vi "EXA_RBW.vi"(0 "VISA resource name":refnum<visa-resource-name>, 5 "Mode":enum16{"Set", "Get"}(ring), 7 "Units":enum16{"Hz", "kHz", "MHz", "GHz"}(ring), 9 "RBW":dbl, 11 "error in":errorcluster) -> (4 "VISA resource name":refnum<visa-resource-name>, 6 "RBW(Hz)":dbl, 15 "error out":errorcluster)   [LabVIEW 2016]
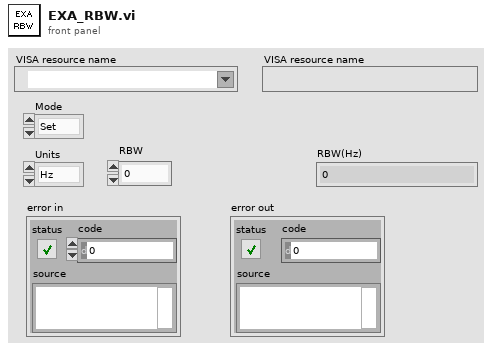
[diagram p1: front panel]
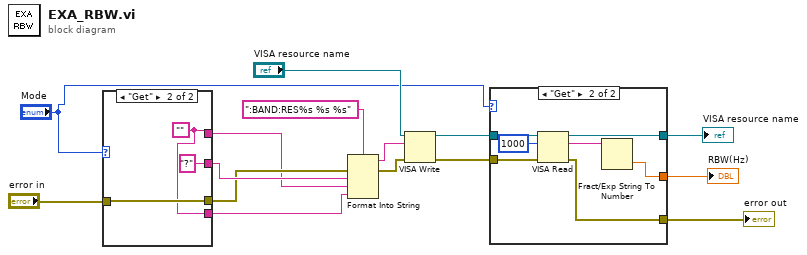
[diagram p0: block diagram]
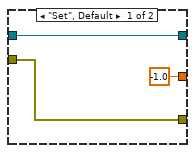
[diagram p2: hidden frame]
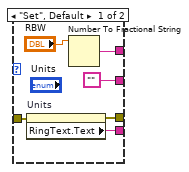
[diagram p3: hidden frame]
diagram:
  n1 = case shown="\"Get\"" "Mode" {
    tunnel: [w16 w22] -> w1
    tunnel: [w21 w22] -> w2
    tunnel: "error in" -> [w20 w23]
    tunnel: [w19 w23] -> w3
    tunnel: ["" "?"] -> w4
    frame "Set", Default {
      n2 = property on="Units" class="Enum (strict)"(error in=w20) -> (error out=w19:errorcluster, "RingText.Text"=w21:string)  [unwired: 1 in, 1 out]
      n3 = Number To Fractional String(number="RBW") -> (F-format string=w16:string)  [unwired: 3 in]
    }
    frame "Get" {
      w22 = ""
    }
  }
  n4 = Format Into String(format string=":BAND:RES%s %s %s", error in=w3, w4, w1, w2) -> (resulting string=w12:string, error out=w14:errorcluster)  [unwired: 1 in]
  n5 = VISA Write(VISA resource name="VISA resource name", write buffer=w12, error in (no error)=w14) -> (VISA resource name out=w8:refnum<visa-resource-name>, error out=w9:errorcluster)  [unwired: 1 out]
  n6 = case shown="\"Get\"" "Mode" {
    tunnel: w9 -> [w25 w34]
    tunnel: w8 -> [w27 w33]
    tunnel: [w27 w32] -> w5
    tunnel: [-1.0 w30] -> w7
    tunnel: [w25 w29] -> w6
    frame "Set", Default {
    }
    frame "Get" {
      n7 = VISA Read(VISA resource name=w33, byte count=u32 1000, error in (no error)=w34) -> (VISA resource name out=w32:refnum<visa-resource-name>, read buffer=w31:string, error out=w29:errorcluster)  [unwired: 1 out]
      n8 = Fract/Exp String To Number(string=w31) -> (number=w30:dbl)  [unwired: 3 in, 1 out]
    }
  }
  "error out" <- w6
  "VISA resource name" <- w5
  "RBW(Hz)" <- w7
